vi "Xs.vi"(1 "Vehicle Frontal Area (Am)":dbl, 2 "Turn-table Centre (Xm)":dbl, 3 "Vehicle Length (Lm)":dbl) -> (0 "Nozzle-source point (Xs)":dbl)   [LabVIEW 2017]
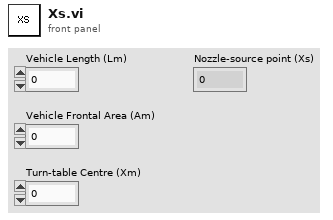
[diagram p1: front panel]
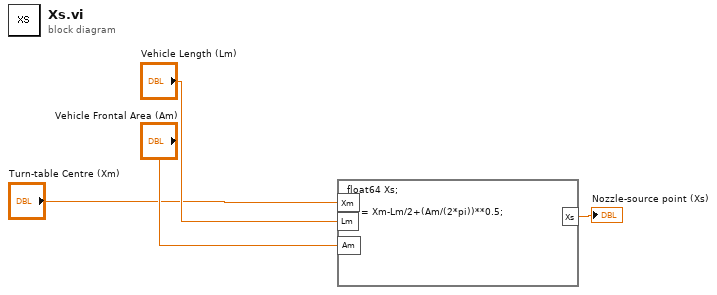
[diagram p0: block diagram]
diagram:
  n1 = formula code="float64 Xs;\n\nXs = Xm-Lm/2+(Am/(2*pi))**0.5;"("Xm"="Turn-table Centre (Xm)", "Lm"="Vehicle Length (Lm)", "Am"="Vehicle Frontal Area (Am)") -> ("Xs"=→"Nozzle-source point (Xs)":dbl)
